vi "Global_ACT_Data Out.vi"() -> ()   [LabVIEW 2023, in "Template_ACT.lvlib"]
uses:
  Template_ACT.lvlib
panel:
  in  "ACT_Template_DBLDataIn":dbl
  in  "ACT_Template_CycleTime(S)":dbl
  in  "ACT_Template_DBLDataOut":dbl
  # "The Names of the Data items in the Global Variable MUST describe who the Single Writer is\nFor Actuator Globals the the naming convention is\n   \nACT_Lib Name_Data Name\n\nExamples:\nACT_Drive_X axis\nACT_Hopper_AgitatorSpeed"
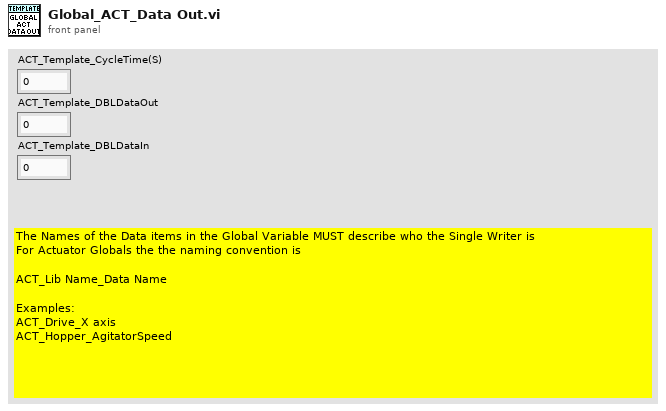
[diagram p1: front panel]
diagram:
